vi "Stage Controller.vi"(8 "Obs Distances Measure Array":dbl[](array[numeric]), 9 "Posture In":dbl[](array[numeric]), 10 "Robot Frame (World)":cluster{"X":sgl, "Y":sgl, "Theta":dbl}, 11 "Start!":bool) -> (2 "Frame Velocity":dbl[](array[numeric]), 3 "Current State":string="Next Goal")   [LabVIEW 2016]
uses:
  StageControl.ctl
panel:
  out "Current State 2":string="Next Goal"
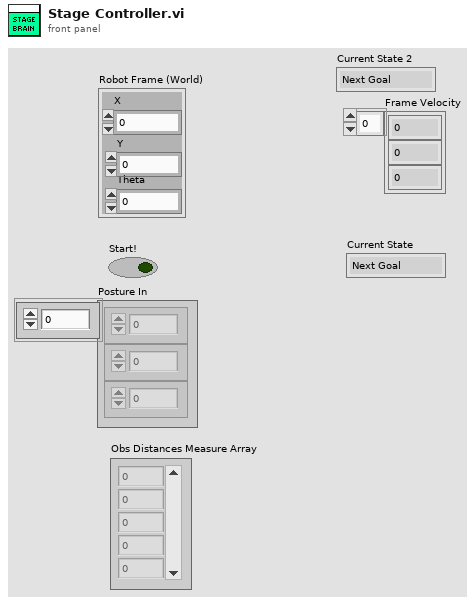
[diagram p1: front panel]
types:
  T1 = typedef "StageControl.ctl" = enum16{"Start", "Stage1", "Stage2", "Stage3", "Stop"}
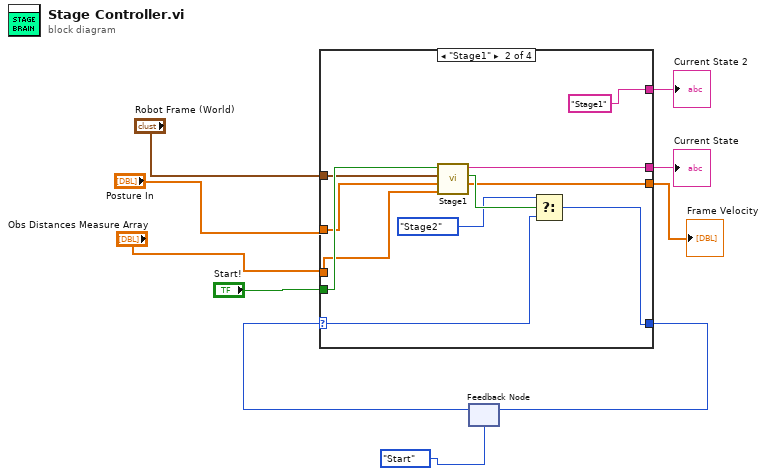
[diagram p0: block diagram]
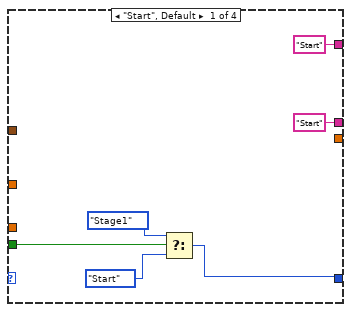
[diagram p2: hidden frame]
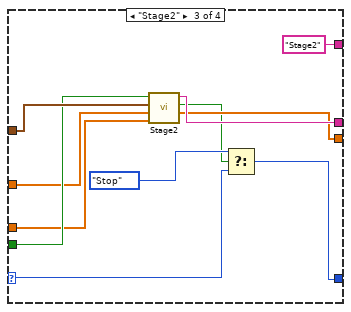
[diagram p3: hidden frame]
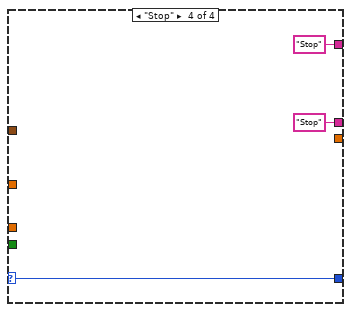
[diagram p4: hidden frame]
diagram:
  n1 = feedback #1(StageControl."Start") -> (w9:T1)
  n2 = case shown="\"Stage1\"" w9 {
    selector: w9 -> [_ w23 w37 w41]
    tunnel: [w13 w24 w36 w41] -> w10
    tunnel: "Start!" -> [w16 w27 w34 _]
    tunnel: ["Start" ("Current State") w22 w33 "Stop" ("Current State")] -> w6
    tunnel: "Robot Frame (World)" -> [_ w21 w35 _]
    tunnel: [_ w20 w32 _] -> w4
    tunnel: ["Start" ("Current State 2") "Stage1" ("Current State 2") "Stage2" ("Current State 2") "Stop" ("Current State 2")] -> w3
    tunnel: "Posture In" -> [_ w18 w29 _]
    tunnel: "Obs Distances Measure Array" -> [_ w17 w28 _]
    frame "Start", Default {
      n3 = Select(t=StageControl."Stage1", s=w16, f=StageControl."Start") -> (s? t:f=w13:T1)
    }
    frame "Stage1" {
      n4 = call "Stage1.vi"("Obs Distances Measure Array"=w17, "Posture In"=w18, "Robot Frame (World)"=w21, "Start"=w27) -> ("Frame Velocity"=w20:dbl[], "Finish Stage?"=w26:bool, "Current State"=w22:string)  [unwired: 5 in]
      n5 = Select(t=StageControl."Stage2", s=w26, f=w23) -> (s? t:f=w24:T1)
    }
    frame "Stage2" {
      n6 = call "Stage2.vi"("Obs Distances Measure Array"=w28, "Posture In"=w29, "Robot Frame (World)"=w35, "Start"=w34) -> ("Frame Velocity"=w32:dbl[], "Finish Stage?"=w31:bool, "Current State"=w33:string)  [unwired: 5 in]
      n7 = Select(t=StageControl."Stop", s=w31, f=w37) -> (s? t:f=w36:T1)
    }
    frame "Stop" {
    }
  }
  "Current State" <- w6
  "Frame Velocity" <- w4
  "Current State 2" <- w3
  n8 = feedback-in #1(w10) -> ()
